vi "ReadTriggerCountNode.vi"(8 "Error In":errorcluster, 11 "Trigger Node In":refnum<k20>) -> (0 "Error Out":errorcluster, 1 "Infinite?":bool, 2 "Count":u32, 3 "Trigger Node Out":refnum<k20>)   [LabVIEW 2012]
uses:
  <vilib>/xml/NI_XML.lvlib
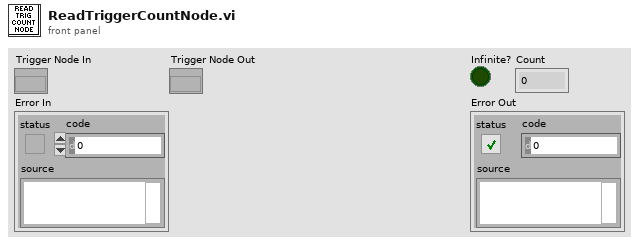
[diagram p1: front panel]
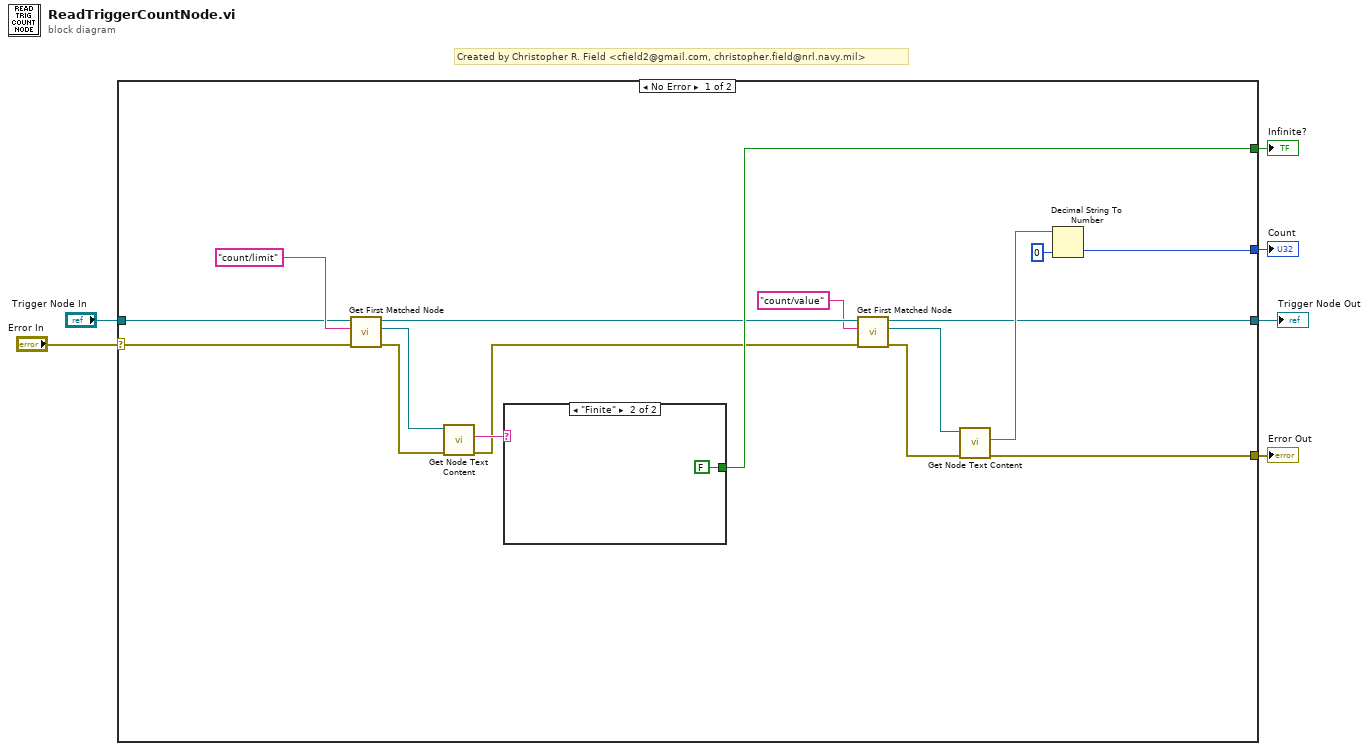
[diagram p0: block diagram]
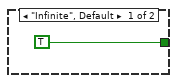
[diagram p2: hidden frame]
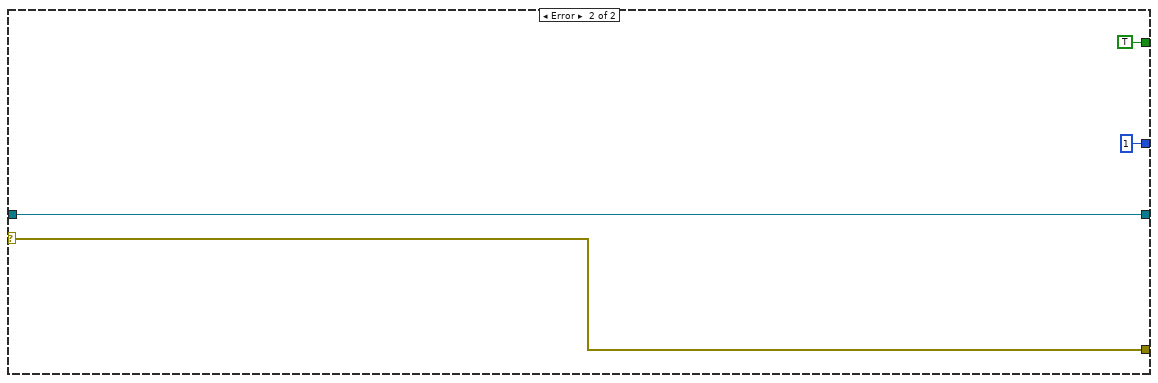
[diagram p3: hidden frame]
diagram:
  # "Created by Christopher R. Field <cfield2@gmail.com, christopher.field@nrl.navy.mil>"
  n1 = case shown="No Error" "Error In" {
    selector: "Error In" -> [w9 w29]
    tunnel: "Trigger Node In" -> [w10 w26]
    tunnel: [w19 TRUE] -> w4
    tunnel: [w11 u32 1] -> w3
    tunnel: [w8 w26] -> w2
    tunnel: [w7 w29] -> w1
    frame No Error {
      n2 = call <vilib>:"Get First Matched Node.vi"("error in (no error)"=w9, "XPath expression"="count/limit", "node in"=w10) -> ("error out"=w21:errorcluster, "node result"=w22:refnum<k20>, "node out"=w18:refnum<k20>)  [unwired: 6 in]
      n3 = call <vilib>:"Get Node Text Content.vi"("error in (no error)"=w21, "node in"=w22) -> ("error out"=w16:errorcluster, "node text"=w20:string)  [unwired: 7 in, 1 out]
      n4 = case shown="\"Finite\"" w20 {
        tunnel: [TRUE FALSE] -> w19
        frame "Infinite", Default {
        }
        frame "Finite" {
        }
      }
      n5 = call <vilib>:"Get First Matched Node.vi"("error in (no error)"=w16, "XPath expression"="count/value", "node in"=w18) -> ("error out"=w14:errorcluster, "node result"=w15:refnum<k20>, "node out"=w8:refnum<k20>)  [unwired: 6 in]
      n6 = call <vilib>:"Get Node Text Content.vi"("error in (no error)"=w14, "node in"=w15) -> ("error out"=w7:errorcluster, "node text"=w13:string)  [unwired: 7 in, 1 out]
      n7 = Decimal String To Number(string=w13, default (0L)=u32 0 ("default (0 I32)")) -> (number=w11:u32)  [unwired: 1 in, 1 out]
    }
    frame Error {
    }
  }
  "Infinite?" <- w4
  "Count" <- w3
  "Trigger Node Out" <- w2
  "Error Out" <- w1
